vi "Launch New Chat Window.vi"(8 "error in (no error)":errorcluster, 11 "Chat Server in":refnum<class "Chat Server.lvclass">) -> (0 "error out":errorcluster, 3 "Chat Server out":refnum<class "Chat Server.lvclass">)   [LabVIEW 2021, in "Chat Server.lvlib" / "Chat Server.lvclass"]
uses:
  Chat Server.lvclass
  C:/Program Files (x86)/National Instruments/LabVIEW 2021/vi.lib/ActorFramework/Actor/Actor.lvclass
  Chat Room Model/Chat Room Model/Chat Room Model.lvclass
  Chat Server.lvclass/Chat Server.ctl
  <vilib>/ActorFramework/Actor/Actor.lvclass
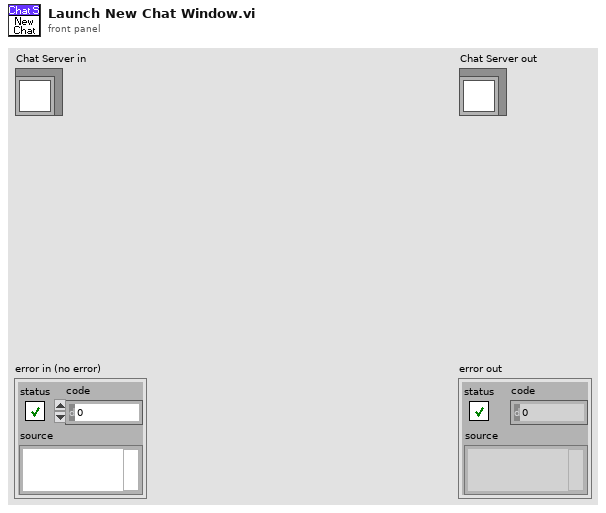
[diagram p1: front panel]
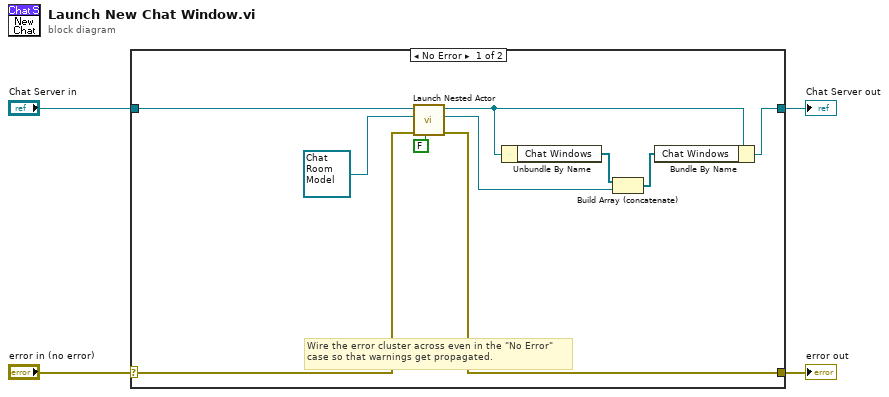
[diagram p0: block diagram]
diagram:
  n1 = case shown="No Error" "error in (no error)" {
    selector: "error in (no error)" -> [w13 w16]
    tunnel: [w12 w16] -> w3
    tunnel: [w9 w15] -> w1
    tunnel: "Chat Server in" -> [w14 w15]
    frame No Error {
      # "Wire the error cluster across even in the \"No Error\"\ncase so that warnings get propagated."
      n2 = call <vilib>:"Launch Nested Actor.vi"("Open Actor Core front panel? (F)"=FALSE, "error in (no error)"=w13, "Nested Actor"=refnum<class "Chat Room Model.lvclass"> refnum ("Chat Room Model.lvlib:Chat Room Model.lvclass"), "Caller Actor in"=w14) -> ("error out"=w12:errorcluster, "Nested Actor's Enqueuer"=w6:refnum<class "Message Enqueuer.lvclass">, "Caller Actor out"=w10:refnum<class "Chat Server.lvclass">)  [unwired: 5 in]
      n3 = Unbundle By Name(w10) -> ("Chat Windows"=w8:refnum<class "Message Enqueuer.lvclass">[])
      n4 = Build Array (concatenate)(w8, w6) -> (w7:refnum<class "Message Enqueuer.lvclass">[])
      n5 = Bundle By Name(cluster=w10, "Chat Windows"=w7) -> (w9:refnum<class "Chat Server.lvclass">)
    }
    frame Error {
    }
  }
  "error out" <- w3
  "Chat Server out" <- w1
